vi "PPMS_Wait.vi"(6 "error in (no error)":errorcluster, 7 "Index":i8) -> (0 "error out":errorcluster, 2 "resulting string 1":string="Wait for Temperature, Timeout 300sec, Continue", 3 "Cancelled?":bool)   [LabVIEW 2017]
doc: "Use this template to create a dialog box. This template polls the state of the buttons on the front panel and does not use events. Use the Dialog Using Events template (not available in Base package) to create a dialog box with event handling."
panel:
  in  "On timeout":i32(ring) items=["Continue", "Abort "]
  in  "Field":bool caption="Wait magnetic field stable"
  in  "Temperature":bool=TRUE caption="Wait temperature stable"
  in  "Timeout(s)":i16=300
  in  "Cancel":bool
  in  "OK":bool
  # "Octubre 2019 V1.2  a-sslcdms"
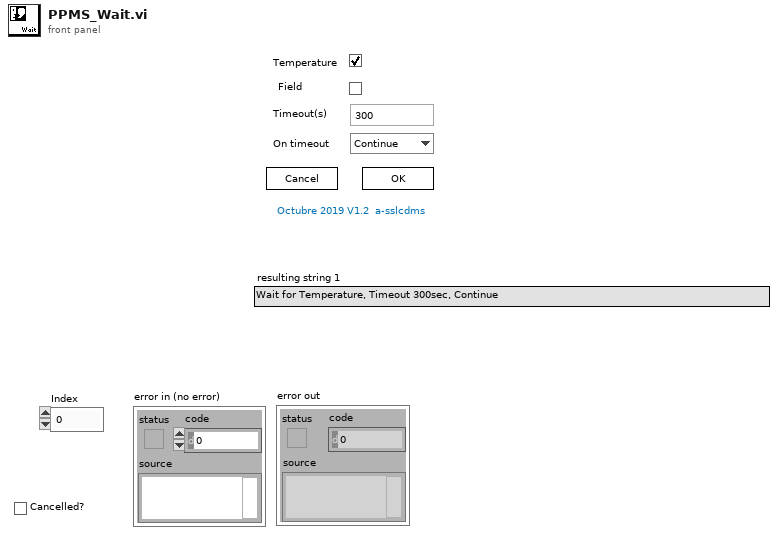
[diagram p1: front panel]
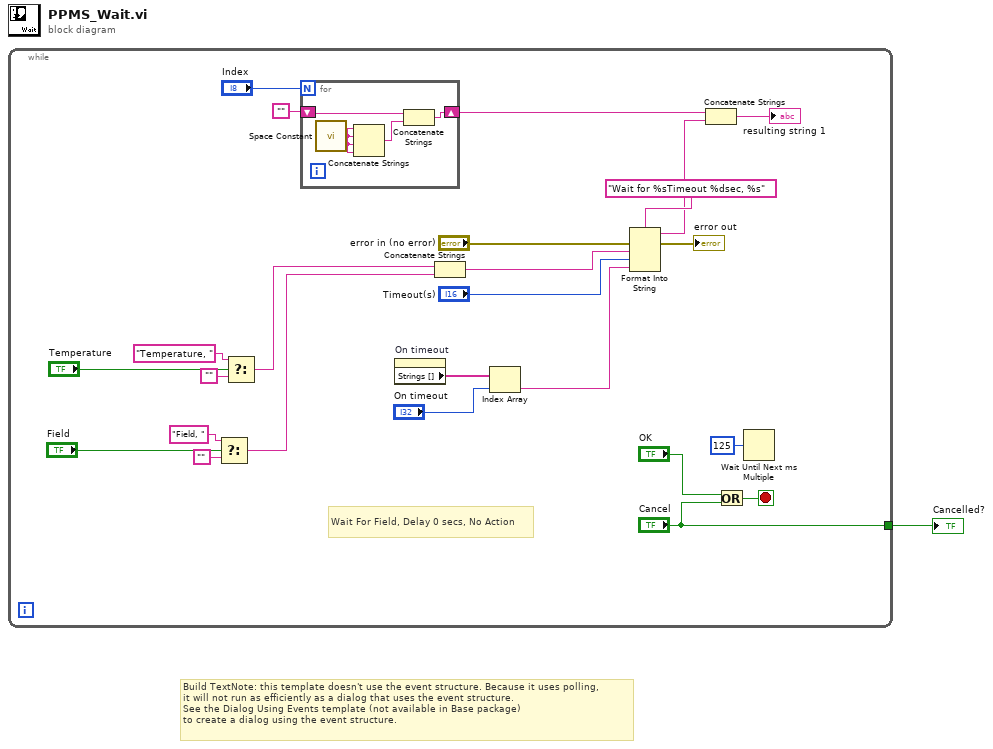
[diagram p0: block diagram]
diagram:
  # "Build TextNote: this template doesn't use the event structure. Because it uses polling, \nit will not run as efficiently as a dialog that uses the event structure.\nSee the Dialog Using Events template (not available in Base package) \nto create a dialog using the event structure."
  n1 = while {
    tunnel: ["Cancel"] -> w1
    stop <- w25 stop-if-true
    # "Wait For Field, Delay 0 secs, No Action"
    n2 = Select(t="Field, " ("format string"), s="Field", f="") -> (s? t:f=w2:string)
    n3 = Select(t="Temperature, " ("format string"), s="Temperature", f="") -> (s? t:f=w3:string)
    n4 = for {
      N: "Index" -> [_]
      shift-right: [w29] -> w15
      shift-left: "" -> [w28]
      n5 = call <vilib>:"Space Constant.vi"() -> ("String"=w27:string)
      n6 = Concatenate Strings(w27, w27, w27, w27) -> (w30:string)
      n7 = Concatenate Strings(w28, w30) -> (w29:string)
    }
    n8 = property on="On timeout" class="Ring (strict)"() -> ("Strings []"=w13:string[])  [unwired: 2 in, 2 out]
    n9 = Concatenate Strings(w3, w2) -> (w10:string)
    n10 = Index Array(array=w13, index="On timeout") -> (element=w11:string)
    n11 = Format Into String(format string="Wait for %sTimeout %dsec, %s", error in="error in (no error)", w10, "Timeout(s)", w11) -> (resulting string=w17:string, error out=→"error out":errorcluster)  [unwired: 1 in]
    n12 = Concatenate Strings(w15, w17) -> (→"resulting string 1":string)
    n13 = Or(x="OK", y="Cancel") -> (x .or. y?=w25:bool)
    n14 = Wait Until Next ms Multiple(millisecond multiple=u32 125) -> ()  [unwired: 1 out]
  }
  "Cancelled?" <- w1
